vi "niRFSysCalReader Fetch Cal Points.vi"(8 "error in":errorcluster, 11 "niRFSysCalReader Handle":T2) -> (0 "error out":errorcluster, 2 "Cal Points":T1(array[cluster]), 3 "niRFSysCalReader Handle out":T2)   [LabVIEW 2018, in "niRFSysCalReader.lvlib"]
doc: "Returns the cal points (i.e. sets of frequency and power / ref level) in the niRFSysCalReader Handle"
uses:
  niRFSysCalReader.lvlib
  INCLUDES/niRFSysCalReader Handle.ctl
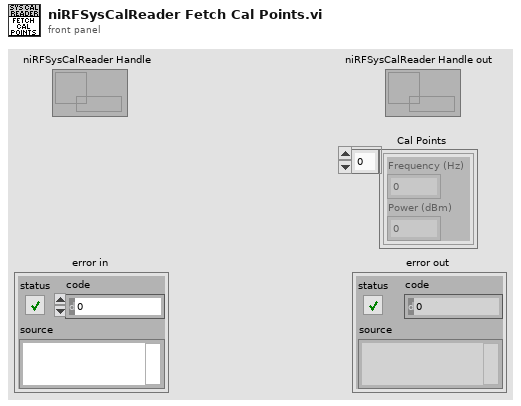
[diagram p1: front panel]
types:
  T1 = cluster{"Frequency (Hz)":dbl, "Power (dBm)":dbl}[]
  T2 = typedef "niRFSysCalReader.lvlib/niRFSysCalReader Handle.ctl" = refnum<data-value>
  T3 = cluster{"Frequency (Hz)":bool, "Power (dBm)":bool}
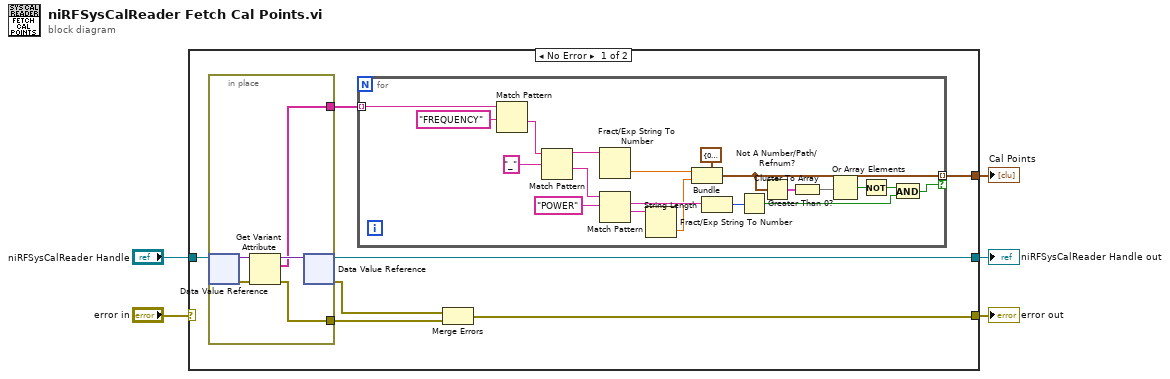
[diagram p0: block diagram]
diagram:
  n1 = case shown="No Error" "error in" {
    selector: "error in" -> [_ w39]
    tunnel: [w12 w38] -> w5
    tunnel: "niRFSysCalReader Handle" -> [w11 w38]
    tunnel: [w10 w39] -> w2
    tunnel: [w6 _] -> w1
    frame No Error {
      n2 = in-place {
        in-place-border: [w35] -> w8
        in-place-border: [w33] -> w7
        n3 = in-place-dvr #1(w11) -> (w37:variant, w34:errorcluster)
        n4 = Get Variant Attribute(Variant=w37, error in=w34) -> (duplicate Variant=w36:variant, names=w33:string[], error out=w35:errorcluster)  [unwired: 2 in, 1 out]
        n5 = in-place-dvr #1(w36) -> (w12:T2, w9:errorcluster)
      }
      n6 = for {
        tunnel: w7 -> [w26] mode=indexing
        tunnel: [w19] -> w6 mode=indexing if=w14
        n7 = Match Pattern(string=w26, regular expression="FREQUENCY" ("string")) -> (after substring=w32:string)  [unwired: 1 in, 3 out]
        n8 = Match Pattern(string=w32, regular expression="_" ("string")) -> (before substring=w31:string, after substring=w30:string)  [unwired: 1 in, 2 out]
        n9 = Fract/Exp String To Number(string=w31) -> (number=w22:dbl)  [unwired: 3 in, 1 out]
        n10 = Match Pattern(string=w30, regular expression="POWER" ("string")) -> (match substring=w28:string, after substring=w29:string)  [unwired: 1 in, 2 out]
        n11 = Fract/Exp String To Number(string=w29) -> (number=w21:dbl)  [unwired: 3 in, 1 out]
        n12 = Bundle(cluster=cluster{"Frequency (Hz)":dbl, "Power (dBm)":dbl} {"Frequency (Hz)"=0.0, "Power (dBm)"=0.0}, "Frequency (Hz)"=w22, "Power (dBm)"=w21) -> (w19:cluster{"Frequency (Hz)":dbl, "Power (dBm)":dbl})
        n13 = String Length(string=w28) -> (length=w27:i32)
        n14 = Greater Than 0?(x=w27) -> (x > 0?=w13:bool)
        n15 = Not A Number/Path/Refnum?(number/path/refnum=w19) -> (NaN/Path/Refnum?=w18:T3)
        n16 = Cluster To Array(cluster=w18) -> (array=w17:bool[])
        n17 = Or Array Elements(Boolean array=w17) -> (logical OR=w16:bool)
        n18 = Not(x=w16) -> (.not. x?=w15:bool)
        n19 = And(x=w15, y=w13) -> (x .and. y?=w14:bool)
      }
      n20 = Merge Errors(w9, w8) -> (w10:errorcluster)
    }
    frame Error {
    }
  }
  "niRFSysCalReader Handle out" <- w5
  "error out" <- w2
  "Cal Points" <- w1
